vi "InfluxDB v2.x Client.vi"(7 "Influx Command":T5, 8 "error in":errorcluster, 9 "Write Data":T1={"Bucket"="", "Timestamp precision"=enum."Seconds", "Line protocol"="", "Measurement"=""}, 10 "Query Data":string, 11 "DataBase Data":T3) -> (0 "error out":errorcluster, 3 "Header-Body Data":T4)   [LabVIEW 2020, in "InfluxDB v2 Client.lvlib"]
doc: "LabVIEW client for InfluDB v2.x"
uses:
  InfluxDB v2 Client.lvlib
  Influx Command.ctl
  Header-Body Data.ctl
  DataBase Data.ctl
  Write Data.ctl
  Write Precision.ctl
  <vilib>/httpClient/POSTBuffer.vi
  <vilib>/httpClient/LabVIEWHTTPClient.lvlib
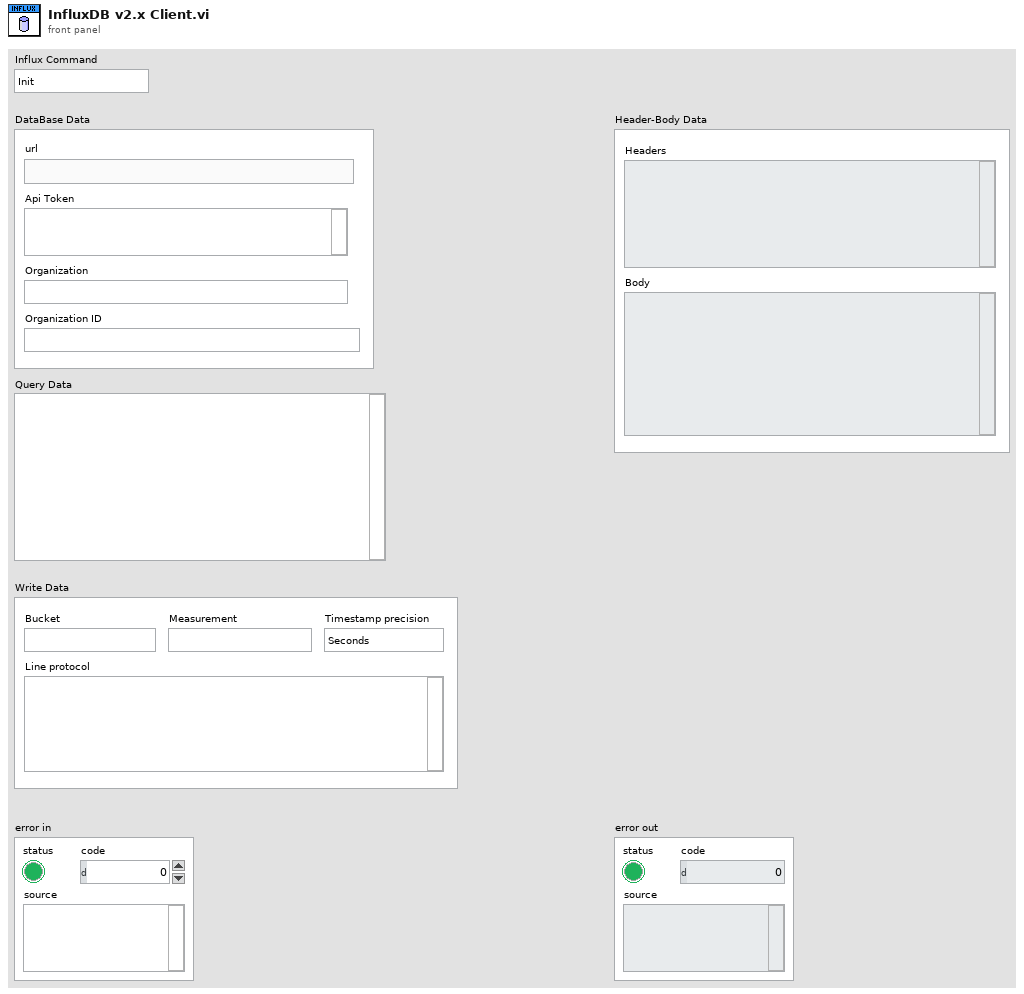
[diagram p1: front panel]
types:
  T1 = typedef "InfluxDB v2 Client.lvlib/Write Data.ctl" = cluster{"Bucket":string, "Timestamp precision":T2, "Line protocol":string, "Measurement":string}
  T2 = typedef "InfluxDB v2 Client.lvlib/Write Precision.ctl" = enum16{"Nanoseconds", "Microseconds", "Milliseconds", "Seconds"}
  T3 = typedef "InfluxDB v2 Client.lvlib/DataBase Data.ctl" = cluster{"Api Token":string, "Organization":string, "url":string, "Organization ID":string}
  T4 = typedef "InfluxDB v2 Client.lvlib/Header-Body Data.ctl" = cluster{"Headers":string, "Body":string}
  T5 = typedef "InfluxDB v2 Client.lvlib/Influx Command.ctl" = enum16{"Init", "Check Auth", "Query Data", "Query ZIP Data", "Write Data", "Close"}
  T6 = typedef "LabVIEWHTTPClient.lvlib/ClientHandle.ctl" = refnum<k1>
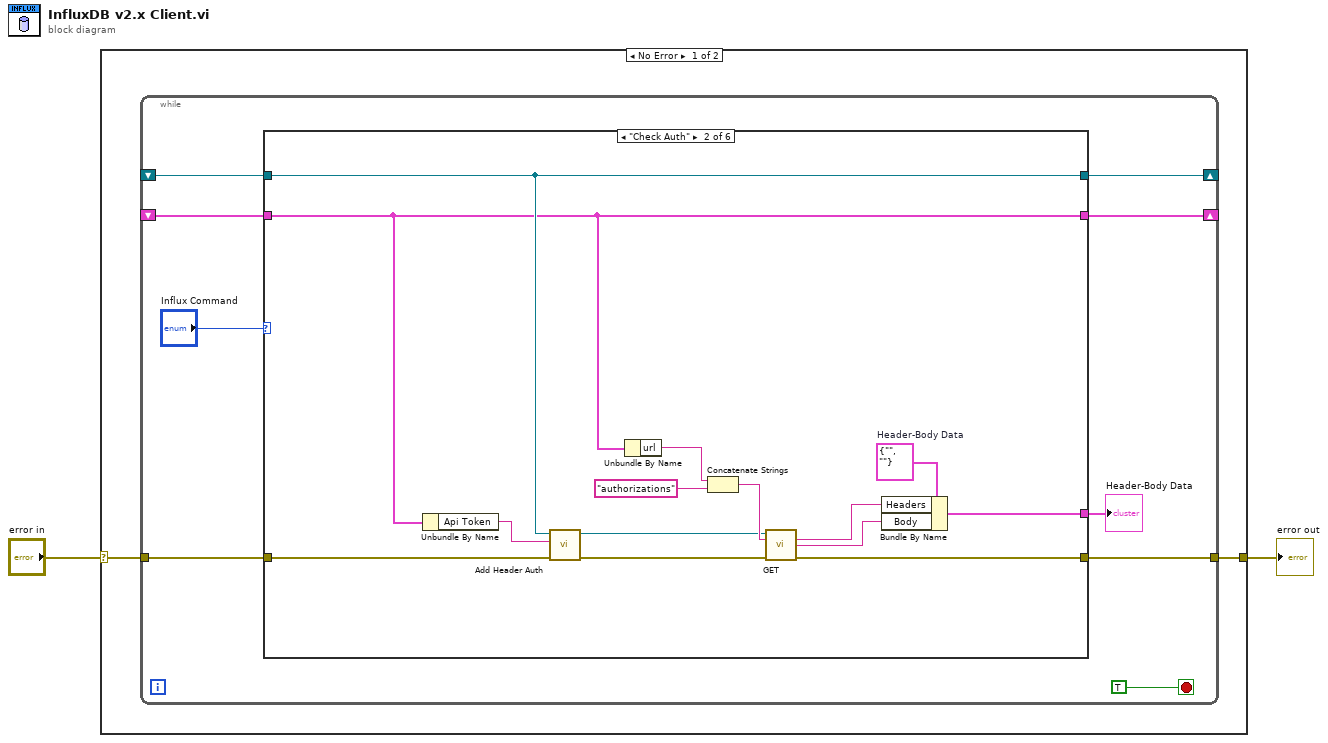
[diagram p0: block diagram]
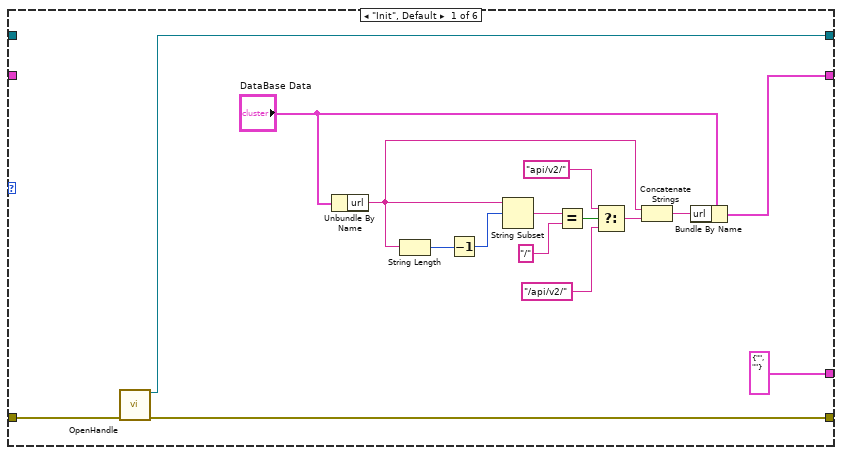
[diagram p2: hidden frame]
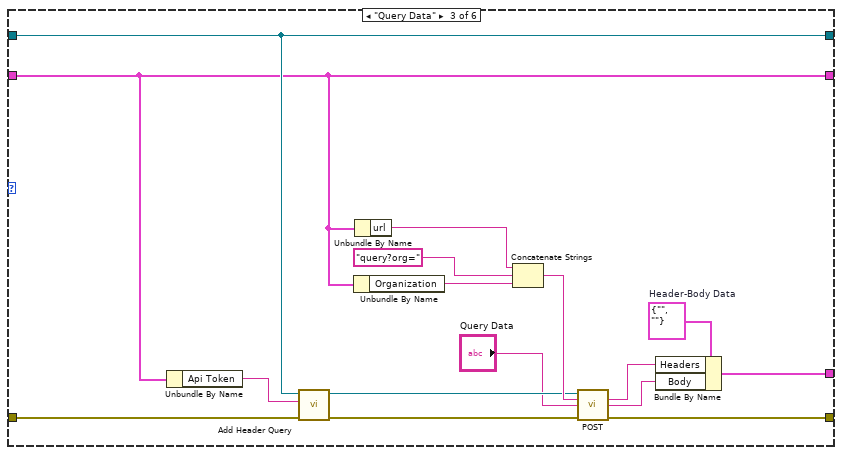
[diagram p3: hidden frame]
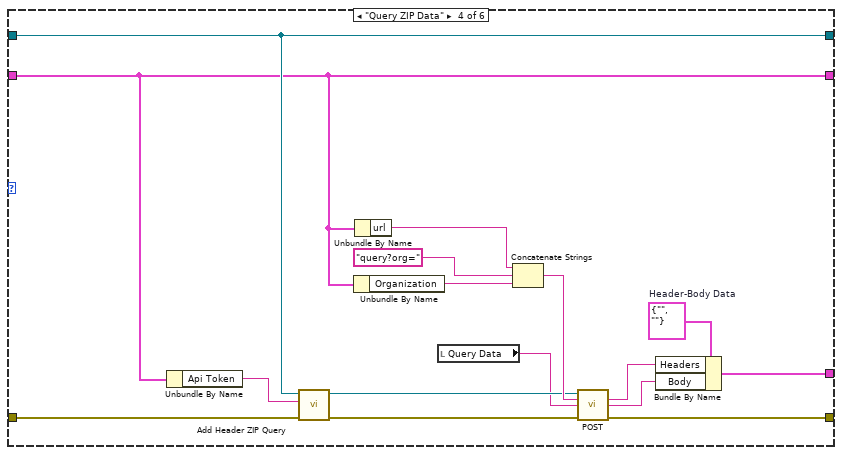
[diagram p4: hidden frame]
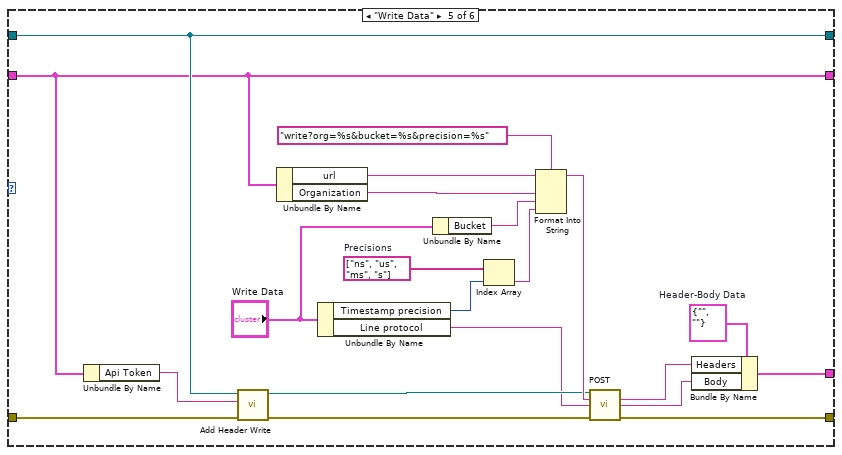
[diagram p5: hidden frame]
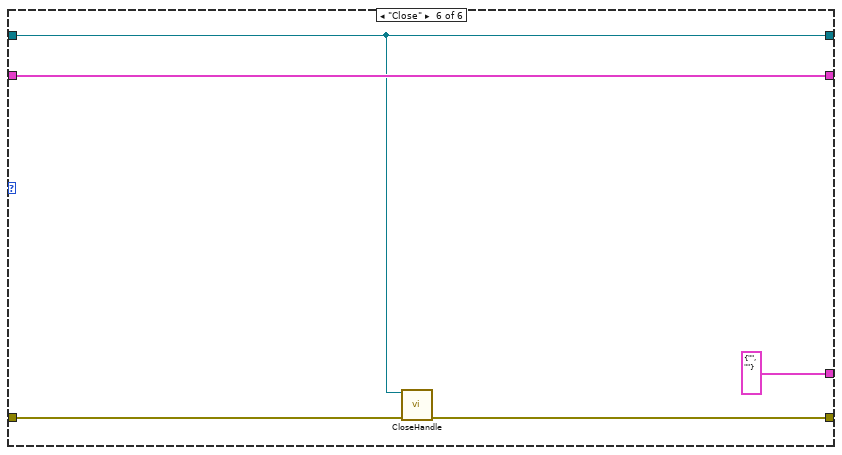
[diagram p6: hidden frame]
diagram:
  n1 = case shown="No Error" "error in" {
    selector: "error in" -> [w4 w102]
    tunnel: [w3 w102] -> w1
    frame No Error {
      n2 = while {
        shift-right: [w11] -> _
        shift-left: _ -> [w10]
        tunnel: w4 -> [w9]
        tunnel: [w8] -> w3
        shift-right: [w7] -> _
        shift-left: _ -> [w6]
        stop <- TRUE stop-if-true
        n3 = case shown="\"Check Auth\"" "Influx Command" {
          tunnel: [w14 w31 w44 w61 w77 w98] -> w11
          tunnel: w10 -> [_ w31 w44 w61 w77 w98]
          tunnel: w9 -> [w26 w34 w47 w64 w80 w101]
          tunnel: [w29 w43 w57 w73 w90 w100] -> w8
          tunnel: [w28 w32 w50 w66 w83 w97] -> w7
          tunnel: w6 -> [_ w32 w50 w66 w83 w97]
          tunnel: [T4 {"Headers"="", "Body"=""} ("Header-Body Data") w39 w53 w69 w86 T4 {"Headers"="", "Body"=""} ("Header-Body Data")] -> w5
          frame "Init", Default {
            n4 = call <vilib>:"OpenHandle.vi"("error in (no error)"=w26) -> ("client handle out"=w28:T6, "error out"=w29:errorcluster)  [unwired: 13 in]
            n5 = Unbundle By Name("DataBase Data") -> ("url"=w17:string)
            n6 = String Length(string=w17) -> (length=w25:i32)
            n7 = Decrement(x=w25) -> (x-1=w24:i32)
            n8 = String Subset(string=w17, offset (0)=w24) -> (substring=w23:string)  [unwired: 1 in]
            n9 = Equal?(x=w23, y="/") -> (x = y?=w21:bool)
            n10 = Select(t="api/v2/", s=w21, f="/api/v2/") -> (s? t:f=w18:string)
            n11 = Concatenate Strings(w17, w18) -> (w16:string)
            n12 = Bundle By Name(cluster="DataBase Data", "url"=w16) -> (w14:T3)
          }
          frame "Check Auth" {
            w42 = T4 {"Headers"="", "Body"=""}  # Header-Body Data
            n13 = Unbundle By Name(w31) -> ("Api Token"=w33:string)
            n14 = call "Add Header Auth.vi"("error in"=w34, "Api Token"=w33, "client handle in"=w32) -> ("error out"=w36:errorcluster, "client handle out"=w35:T6)  [unwired: 7 in]
            n15 = Unbundle By Name(w31) -> ("url"=w30:string)
            n16 = Concatenate Strings(w30, "authorizations" ("string")) -> (w37:string)
            n17 = call <vilib>:"GET.vi"("client handle"=w35, "url"=w37, "error in (no error)"=w36) -> ("headers"=w41:string, "body"=w40:string, "error out"=w43:errorcluster)  [unwired: 9 in, 1 out]
            n18 = Bundle By Name(cluster=w42, "Headers"=w41, "Body"=w40) -> (w39:T4)
          }
          frame "Query Data" {
            w54 = T4 {"Headers"="", "Body"=""}  # Header-Body Data
            n19 = Unbundle By Name(w44) -> ("Api Token"=w49:string)
            n20 = call "Add Header Query.vi"("error in"=w47, "Api Token"=w49, "client handle in"=w50) -> ("error out"=w52:errorcluster, "client handle out"=w51:T6)  [unwired: 7 in]
            n21 = Unbundle By Name(w44) -> ("Organization"=w45:string)
            n22 = Unbundle By Name(w44) -> ("url"=w46:string)
            n23 = Concatenate Strings(w46, "query?org=", w45) -> (w58:string)
            n24 = call-poly <vilib>:"POST.vi"("client handle"=w51, "url"=w58, "buffer"="Query Data", "error in (no error)"=w52) -> ("headers"=w55:string, "body"=w56:string, "error out"=w57:errorcluster)  [unwired: 8 in, 1 out]
            n25 = Bundle By Name(cluster=w54, "Headers"=w55, "Body"=w56) -> (w53:T4)
          }
          frame "Query ZIP Data" {
            w70 = T4 {"Headers"="", "Body"=""}  # Header-Body Data
            n26 = Unbundle By Name(w61) -> ("Api Token"=w65:string)
            n27 = call "Add Header ZIP Query.vi"("error in"=w64, "Api Token"=w65, "client handle in"=w66) -> ("error out"=w68:errorcluster, "client handle out"=w67:T6)  [unwired: 7 in]
            n28 = Unbundle By Name(w61) -> ("Organization"=w62:string)
            n29 = Unbundle By Name(w61) -> ("url"=w63:string)
            n30 = local read "Query Data"() -> (w60:string)
            n31 = Concatenate Strings(w63, "query?org=", w62) -> (w74:string)
            n32 = call-poly <vilib>:"POST.vi"("client handle"=w67, "url"=w74, "buffer"=w60, "error in (no error)"=w68) -> ("headers"=w71:string, "body"=w72:string, "error out"=w73:errorcluster)  [unwired: 8 in, 1 out]
            n33 = Bundle By Name(cluster=w70, "Headers"=w71, "Body"=w72) -> (w69:T4)
          }
          frame "Write Data" {
            w89 = T4 {"Headers"="", "Body"=""}  # Header-Body Data
            w94 = string[] ["ns", "us", "ms", "s"]  # Precisions
            n34 = Unbundle By Name(w77) -> ("Api Token"=w81:string)
            n35 = call "Add Header Write.vi"("error in"=w80, "Api Token"=w81, "client handle in"=w83) -> ("error out"=w85:errorcluster, "client handle out"=w84:T6)  [unwired: 7 in]
            n36 = Unbundle By Name(w77) -> ("url"=w79:string, "Organization"=w78:string)
            n37 = Unbundle By Name("Write Data") -> ("Timestamp precision"=w92:T2, "Line protocol"=w76:string)
            n38 = Unbundle By Name("Write Data") -> ("Bucket"=w95:string)
            n39 = Index Array(array=w94, index=w92) -> (element=w93:string)
            n40 = Format Into String(format string="write?org=%s&bucket=%s&precision=%s", initial string=w79, w78, w95, w93) -> (resulting string=w91:string)  [unwired: 1 in, 1 out]
            n41 = call-poly <vilib>:"POST.vi"("client handle"=w84, "url"=w91, "buffer"=w76, "error in (no error)"=w85) -> ("headers"=w87:string, "body"=w88:string, "error out"=w90:errorcluster)  [unwired: 8 in, 1 out]
            n42 = Bundle By Name(cluster=w89, "Headers"=w87, "Body"=w88) -> (w86:T4)
          }
          frame "Close" {
            n43 = call <vilib>:"CloseHandle.vi"("client handle"=w97, "error in (no error)"=w101) -> ("error out"=w100:errorcluster)  [unwired: 13 in]
          }
        }
        "Header-Body Data" <- w5
      }
    }
    frame Error {
    }
  }
  "error out" <- w1
